vi "Write Start Camera 2.vi"(8 "error in (no error)":errorcluster, 10 "IMAQdx Session":T1, 11 "HIJ Multiple Cams App Demo in":refnum<class "HIJ 4 Alignment Cams App.lvclass">) -> (0 "error out":errorcluster, 3 "HIJ Multiple Cams App Demo out":refnum<class "HIJ 4 Alignment Cams App.lvclass">)   [LabVIEW 2014, in "HIJ 4 Alignment Cams App.lvlib" / "HIJ 4 Alignment Cams App.lvclass"]
uses:
  HIJ 4 Alignment Cams App.lvclass
  <vilib>/userdefined/High Color/IMAQdx.ctl
  HIJ 4 Alignment Cams App.lvclass/HIJ 4 Alignment Cams App.ctl
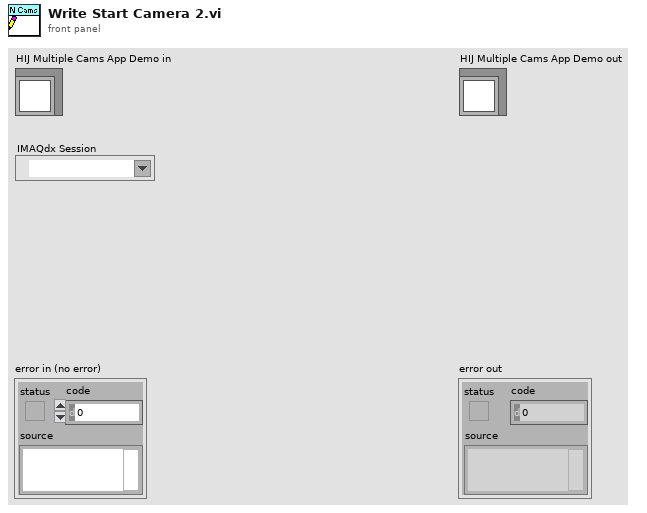
[diagram p1: front panel]
types:
  T1 = typedef "IMAQdx.ctl" = refnum<k21>
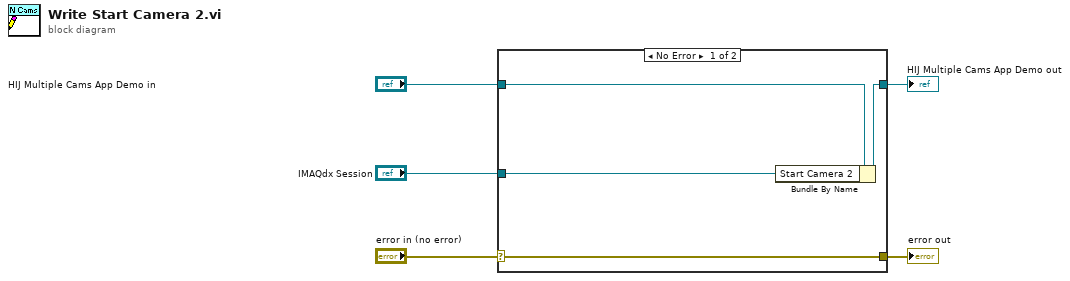
[diagram p0: block diagram]
diagram:
  n1 = case shown="No Error" "error in (no error)" {
    selector: "error in (no error)" -> [w9 w10]
    tunnel: [w9 w10] -> w4
    tunnel: [w7 w11] -> w2
    tunnel: "HIJ Multiple Cams App Demo in" -> [w8 w11]
    tunnel: "IMAQdx Session" -> [w6 _]
    frame No Error {
      n2 = Bundle By Name(cluster=w8, "Start Camera 2"=w6) -> (w7:refnum<class "HIJ 4 Alignment Cams App.lvclass">)
    }
    frame Error {
    }
  }
  "error out" <- w4
  "HIJ Multiple Cams App Demo out" <- w2
